vi "Pre Launch Init.vi"(11 "PredictiveMaintenance in":refnum<class "PredictiveMaintenance.lvclass">) -> (0 "error out":errorcluster, 3 "PredictiveMaintenance out":refnum<class "PredictiveMaintenance.lvclass">)   [LabVIEW 2019, in "PredictiveMaintenance.lvlib" / "PredictiveMaintenance.lvclass"]
doc: "(<B>Filename</B>: Actor Framework.lvlib:Actor.lvclass:Pre Launch Init.vi)\n\nDefines behavior that occurs after the Launch Nested Actor method is invoked but before the actor's Actor Core method begins running.\n\nBy default, this method does nothing. A descendant class may override it to define behavior."
uses:
  PredictiveMaintenance.lvclass
  PredictiveMaintenance.lvclass/PredictiveMaintenance.ctl
  typedefs/EventData.ctl
  typedefs/Trigger_Data.ctl
  <vilib>/ActorFramework/Actor/Actor.lvclass
  ConfigClass/ConfigClass/ConfigClass.lvclass
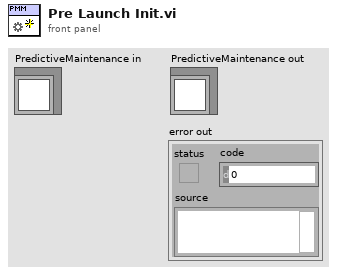
[diagram p1: front panel]
types:
  T1 = typedef "PredictiveMaintenance.lvlib/PredictiveMaintenance.lvclass/Trigger_Data.ctl" = cluster{"trigger":string, "curr_val (h)":dbl, "warn_limit (h)":dbl, "err_limit (h)":dbl, "running_timestamp":timestamp, "counter (h)":dbl}
  T2 = typedef "PredictiveMaintenance.lvlib/PredictiveMaintenance.lvclass/EventData.ctl" = cluster{"event":string, "curr_val":dbl, "warn_limit":dbl, "err_limit":dbl}
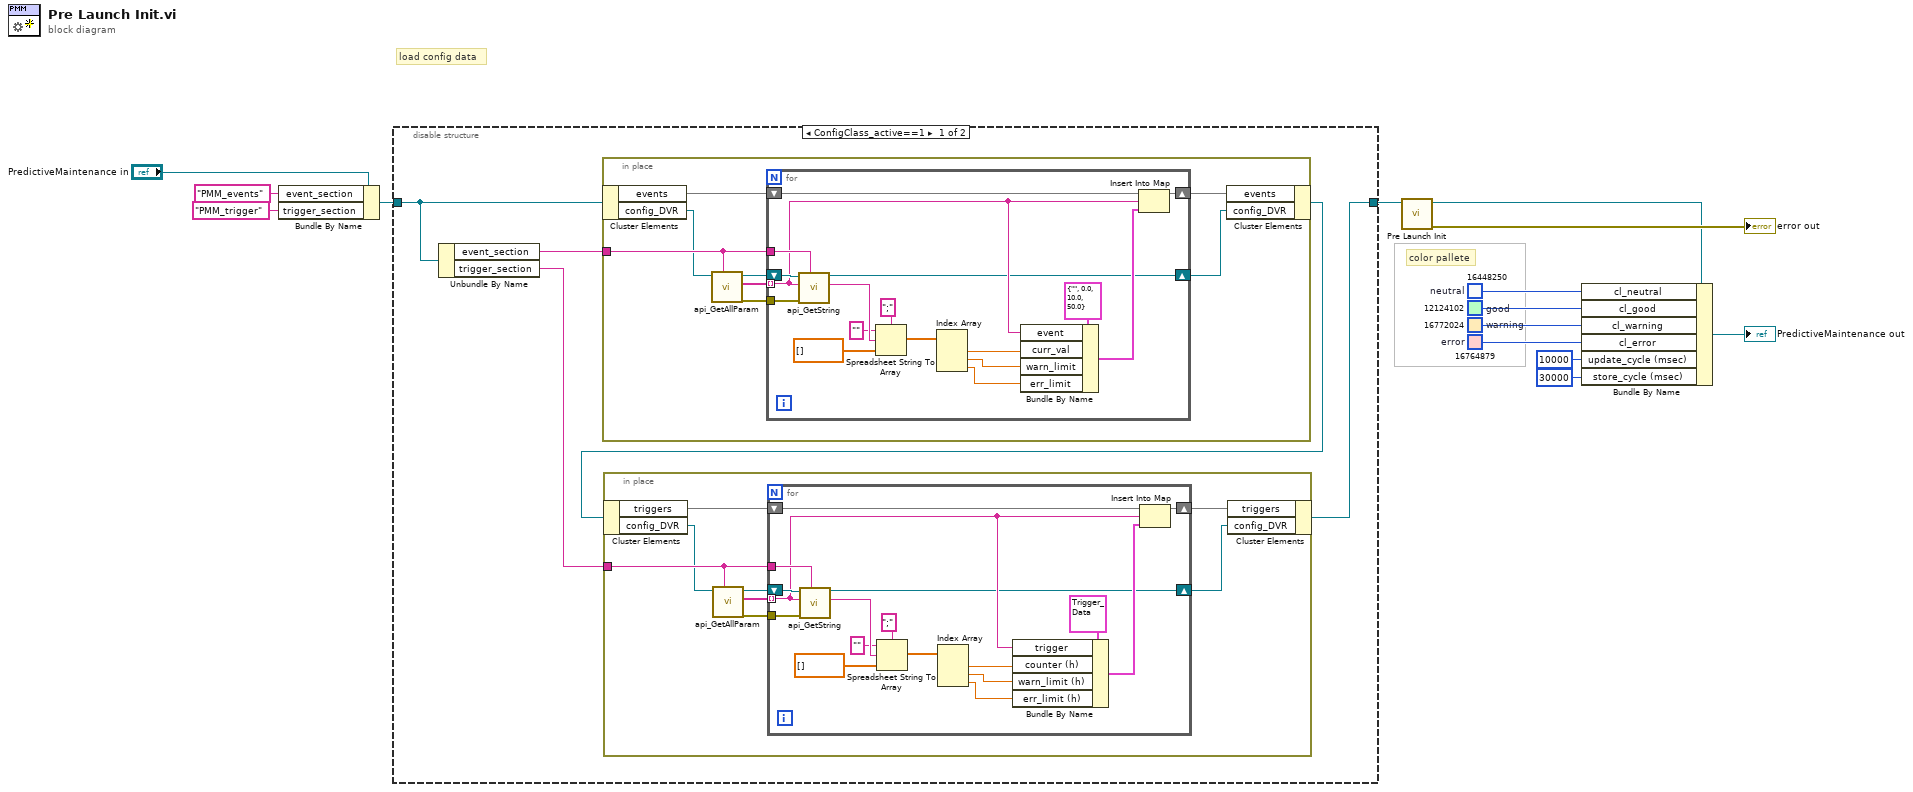
[diagram p0: block diagram]
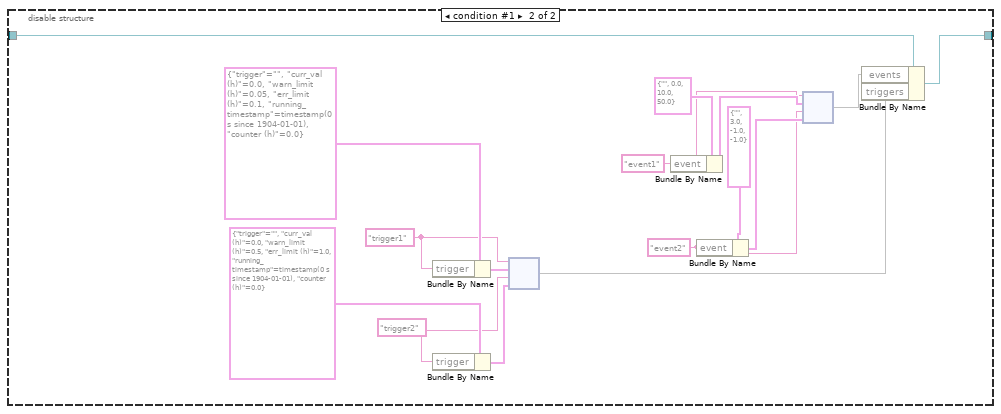
[diagram p2: hidden frame]
diagram:
  w11 = u32 16448250  # neutral
  w9 = u32 16764879  # error
  w8 = u32 16772024  # warning
  w10 = u32 12124102  # good
  # "color pallete"
  # "load config data"
  n1 = Bundle By Name(cluster="PredictiveMaintenance in", "event_section"="PMM_events" ("param_section"), "trigger_section"="PMM_trigger") -> (w5:refnum<class "PredictiveMaintenance.lvclass">)
  n2 = disable-structure shown="ConfigClass_active==1" {
    disable-tunnel: w5 -> [w17 w79]
    disable-tunnel: [w18 w78] -> w4
    frame condition #0 (active) {
      n3 = Unbundle By Name(w17) -> ("event_section"=w16:string, "trigger_section"=w15:string)
      n4 = in-place {
        in-place-border: w16 -> [w51]
        n5 = in-place-cluster #1(w17) -> ("events"=w48:map{string, T2}, "config_DVR"=w46:refnum<data-value>)
        n6 = call "api_GetAllParam.vi"("group"=w51, "ConfigClass_DVR"=w46) -> ("error out"=w49:errorcluster, "params"=w50:string[], "ConfigClass_DVR_out"=w52:refnum<data-value>)  [unwired: 7 in]
        n7 = for {
          tunnel: w51 -> [w68]
          tunnel: w50 -> [w56] mode=indexing
          tunnel: w49 -> [w67]
          shift-right: [w53] -> w45
          shift-left: w52 -> [w69]
          shift-right: [w54] -> w47
          shift-left: w48 -> [w55]
          n8 = call "api_GetString.vi"("group"=w68, "error in (no error)"=w67, "param"=w56, "ConfigClass_DVR"=w69) -> ("string_out"=w65:string, "ConfigClass_DVR_out"=w53:refnum<data-value>)  [unwired: 5 in, 1 out]
          n9 = Spreadsheet String To Array(delimiter (Tab)=";", format string="", spreadsheet string=w65, array type (2D Dbl)=dbl[] []) -> (array=w62:dbl[])
          n10 = Index Array(array=w62) -> (element #1=w61:dbl, element #2=w60:dbl, element #3=w59:dbl)  [unwired: 3 in]
          n11 = Bundle By Name(cluster=T2 {"event"="", "curr_val"=0.0, "warn_limit"=10.0, "err_limit"=50.0} ("event_data"), "event"=w56, "curr_val"=w61, "warn_limit"=w60, "err_limit"=w59) -> (w57:T2)
          n12 = Insert Into Map(map in=w55, key=w56, value=w57) -> (map out=w54:map{string, T2})  [unwired: 2 out]
        }
        n13 = in-place-cluster #1("events"=w47, "config_DVR"=w45) -> (w19:refnum<class "PredictiveMaintenance.lvclass">)
      }
      n14 = in-place {
        in-place-border: w15 -> [w26]
        n15 = in-place-cluster #2(w19) -> ("triggers"=w23:map{string, T1}, "config_DVR"=w21:refnum<data-value>)
        n16 = call "api_GetAllParam.vi"("group"=w26, "ConfigClass_DVR"=w21) -> ("error out"=w24:errorcluster, "params"=w25:string[], "ConfigClass_DVR_out"=w27:refnum<data-value>)  [unwired: 7 in]
        n17 = for {
          tunnel: w26 -> [w43]
          tunnel: w25 -> [w32] mode=indexing
          tunnel: w24 -> [w42]
          shift-right: [w29] -> w20
          shift-left: w27 -> [w44]
          shift-right: [w30] -> w22
          shift-left: w23 -> [w31]
          n18 = call "api_GetString.vi"("group"=w43, "error in (no error)"=w42, "param"=w32, "ConfigClass_DVR"=w44) -> ("string_out"=w40:string, "ConfigClass_DVR_out"=w29:refnum<data-value>)  [unwired: 5 in, 1 out]
          n19 = Spreadsheet String To Array(delimiter (Tab)=";", format string="", spreadsheet string=w40, array type (2D Dbl)=dbl[] []) -> (array=w37:dbl[])
          n20 = Index Array(array=w37) -> (element #1=w36:dbl, element #2=w35:dbl, element #3=w34:dbl)  [unwired: 3 in]
          n21 = Bundle By Name(cluster=T1 {"trigger"="", "curr_val (h)"=0.0, "warn_limit (h)"=-1.0, "err_limit (h)"=-1.0, "running_timestamp"=timestamp(0 s since 1904-01-01), "counter (h)"=0.0} ("event_data"), "trigger"=w32, "counter (h)"=w36, "warn_limit (h)"=w35, "err_limit (h)"=w34) -> (w33:T1)
          n22 = Insert Into Map(map in=w31, key=w32, value=w33) -> (map out=w30:map{string, T1})  [unwired: 2 out]
        }
        n23 = in-place-cluster #2("triggers"=w22, "config_DVR"=w20) -> (w18:refnum<class "PredictiveMaintenance.lvclass">)
      }
    }
    frame condition #1 {
      w73 = "trigger2" ("event")
      w71 = "trigger1" ("event")
      w82 = "event2" ("event")
      w80 = "event1" ("event")
      n24 = Bundle By Name(cluster=T1 {"trigger"="", "curr_val (h)"=0.0, "warn_limit (h)"=0.05, "err_limit (h)"=0.1, "running_timestamp"=timestamp(0 s since 1904-01-01), "counter (h)"=0.0} ("event_data"), "trigger"=w71) -> (w75:T1)
      n25 = Bundle By Name(cluster=T1 {"trigger"="", "curr_val (h)"=0.0, "warn_limit (h)"=0.5, "err_limit (h)"=1.0, "running_timestamp"=timestamp(0 s since 1904-01-01), "counter (h)"=0.0} ("event_data"), "trigger"=w73) -> (w76:T1)
      n26 = node(w71, w75, w73, w76) -> (w70:map{string, T1})
      n27 = Bundle By Name(cluster=T2 {"event"="", "curr_val"=0.0, "warn_limit"=10.0, "err_limit"=50.0} ("event_data"), "event"=w80) -> (w84:T2)
      n28 = Bundle By Name(cluster=T2 {"event"="", "curr_val"=3.0, "warn_limit"=-1.0, "err_limit"=-1.0} ("event_data"), "event"=w82) -> (w85:T2)
      n29 = node(w80, w84, w82, w85) -> (w77:map{string, T2})
      n30 = Bundle By Name(cluster=w79, "events"=w77, "triggers"=w70) -> (w78:refnum<class "PredictiveMaintenance.lvclass">)
    }
  }
  n31 = call-parent "Pre Launch Init.vi"("Actor in"=w4) -> ("error out"=→"error out":errorcluster, "Actor out"=w13:refnum<class "PredictiveMaintenance.lvclass">)  [unwired: 9 in]
  n32 = Bundle By Name(cluster=w13, "cl_neutral"=w11, "cl_good"=w10, "cl_warning"=w8, "cl_error"=w9, "update_cycle (msec)"=10000, "store_cycle (msec)"=30000) -> (→"PredictiveMaintenance out":refnum<class "PredictiveMaintenance.lvclass">)
